vi "DI A Fault Clear.vi"(8 "Device Inputs":dbl[](array[numeric]), 10 "A Fault Clear Indexes":T2) -> (3 "A Fault Clear":T1)   [LabVIEW 2016, in "DCM Engine.lvlib"]
uses:
  DCM Engine.lvlib
  <vilib>/Powertrain Controls/Device Drivers/DCM/Tools/FPGA/8 Channels.ctl
  <vilib>/Powertrain Controls/Device Drivers/DCM/Tools/FPGA/DCM - FPGA - Tools.lvlib
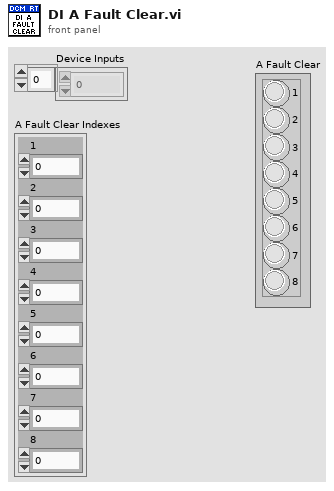
[diagram p1: front panel]
types:
  T1 = typedef "DCM - FPGA - Tools.lvlib/8 Channels.ctl" = cluster{"1":bool, "2":bool, "3":bool, "4":bool, "5":bool, "6":bool, "7":bool, "8":bool}
  T2 = cluster{"1":i32, "2":i32, "3":i32, "4":i32, "5":i32, "6":i32, "7":i32, "8":i32}
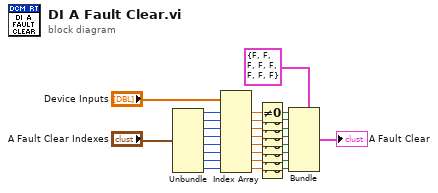
[diagram p0: block diagram]
diagram:
  n1 = Unbundle("A Fault Clear Indexes") -> ("1"=w1:i32, "2"=w8:i32, "3"=w7:i32, "4"=w6:i32, "5"=w5:i32, "6"=w4:i32, "7"=w3:i32, "8"=w2:i32)
  n2 = Index Array(array="Device Inputs", index #1=w1, index #2=w8, index #3=w7, index #4=w6, index #5=w5, index #6=w4, index #7=w3, index #8=w2) -> (element #1=w10:dbl, element #2=w12:dbl, element #3=w13:dbl, element #4=w14:dbl, element #5=w15:dbl, element #6=w16:dbl, element #7=w17:dbl, element #8=w11:dbl)
  n3 = Not Equal To 0?(x=w10) -> (x != 0?=w25:bool)
  n4 = Not Equal To 0?(x=w12) -> (x != 0?=w24:bool)
  n5 = Not Equal To 0?(x=w13) -> (x != 0?=w23:bool)
  n6 = Not Equal To 0?(x=w14) -> (x != 0?=w22:bool)
  n7 = Not Equal To 0?(x=w15) -> (x != 0?=w21:bool)
  n8 = Not Equal To 0?(x=w16) -> (x != 0?=w20:bool)
  n9 = Not Equal To 0?(x=w17) -> (x != 0?=w19:bool)
  n10 = Not Equal To 0?(x=w11) -> (x != 0?=w18:bool)
  n11 = Bundle(cluster=T1 {"1"=FALSE, "2"=FALSE, "3"=FALSE, "4"=FALSE, "5"=FALSE, "6"=FALSE, "7"=FALSE, "8"=FALSE} ("A Fault Clear in"), "1"=w25, "2"=w24, "3"=w23, "4"=w22, "5"=w21, "6"=w20, "7"=w19, "8"=w18) -> (→"A Fault Clear":T1)
